vi "set_behaviour_flag.vi"(6 "timeout (25000ms)":i32=25000, 8 "error in (no error)":errorcluster, 10 "Parameter":T1={"Permenant?"=FALSE, "Word Index"=0, "New Value"=0, "Offset"=0, "data size"=1}, 11 "daemon reference in":refnum<k5>) -> (0 "error out":errorcluster, 2 "response":string, 3 "daemon reference out":refnum<k5>, 5 "command out":string="random")   [LabVIEW 2017]
doc: "<b>Command: </b>\"template\"\n\n<b>Description: </b> This command does something.\n\n<b>Parameters: </b> None\n____________________________________________\nDIPC 692 Daemon API 10.0.0.1\nSam Tee - Dyson Technology Ltd\nCopyright (c) 2024, Dyson Technology Ltd"
panel:
  out "parameter(s) in":string
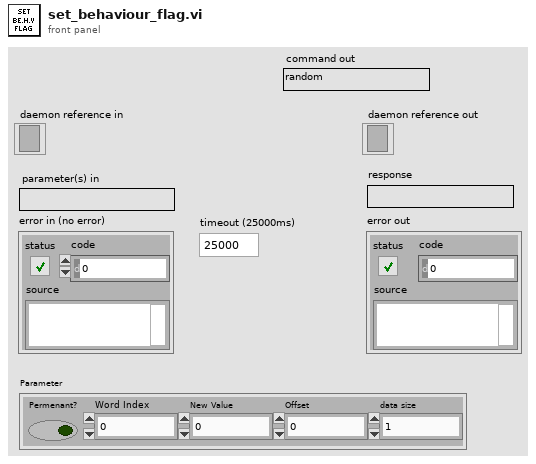
[diagram p1: front panel]
types:
  T1 = cluster{"Permenant?":bool, "Word Index":i64, "New Value":i64, "Offset":i64, "data size":i64}
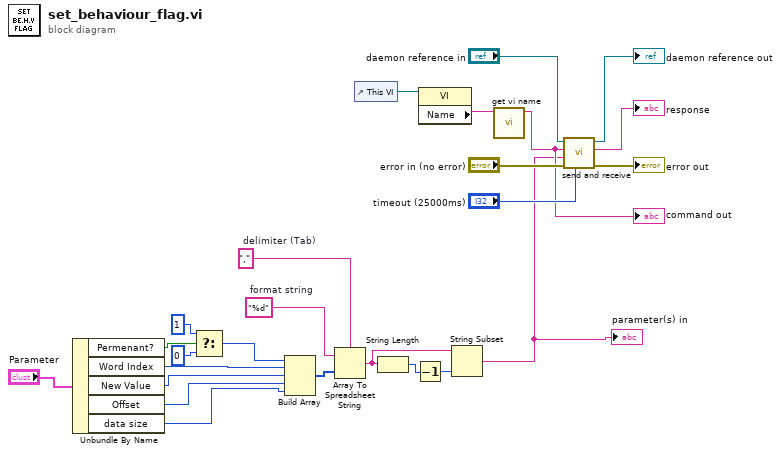
[diagram p0: block diagram]
diagram:
  w13 = ","  # delimiter (Tab)
  w16 = "%d"  # format string
  n1 = Unbundle By Name("Parameter") -> ("Permenant?"=w11:bool, "Word Index"=w7:i64, "New Value"=w3:i64, "Offset"=w2:i64, "data size"=w1:i64)
  n2 = Select(t=1, s=w11, f=0) -> (s? t:f=w8:i32)
  n3 = Build Array(w8, w7, w3, w2, w1) -> (w6:i64[])
  n4 = Array To Spreadsheet String(delimiter (Tab)=w13, array=w6, 3:w16) -> (spreadsheet string=w5:string)
  n5 = control-ref of="This VI"() -> (w19:refnum<vi>)
  n6 = String Length(string=w5) -> (length=w15:i32)
  n7 = Decrement(x=w15) -> (x-1=w14:i32)
  n8 = property class="VI"(reference=w19) -> ("Name"=w18:string)  [unwired: 1 in, 2 out]
  n9 = String Subset(string=w5, length (rest)=w14) -> (substring=w4:string)  [unwired: 1 in]
  "parameter(s) in" <- w4
  n10 = call "get vi name.vi"("library.lvlib:name.vi"=w18) -> ("vi name"=w17:string)  [unwired: 10 in]
  "command out" <- w17
  n11 = call "send and receive.vi"("timeout (25000ms)"="timeout (25000ms)", "error in (no error)"="error in (no error)", "data"=w4, "command"=w17, "daemon reference in"="daemon reference in") -> ("error out"=→"error out":errorcluster, "response"=→"response":string, "daemon reference out"=→"daemon reference out":refnum<k5>)  [unwired: 4 in]
